vi "writePositionFirgelli.vi"(8 "error in (no error)":errorcluster, 9 "lengthMax":dbl=100.0, 10 "Position (mm)":dbl(slide)=1.0 min=0.0 max=100.0 step=0.1 scale=0.0..100.0 scale format="%.2f", 11 "handleIn":u32 format="%x") -> (0 "error out":errorcluster, 2 "regSetting":u16, 3 "handleOut":u32 format="%x")   [LabVIEW 2019]
doc: "0x20 SET_POSITION\nThis command allows USB control and disables RC, I, and V inputs until the system is rebooted. The data sent with this command determines what position the actuator moves too.\n\nFor example, to half way extend(25mm) a 50mm actuator, send 512. (The calculated value is rounded to a whole number).\n\nWritten by: Complete Automated Solutions\nwww.CompleteAutomatedSolutions.com"
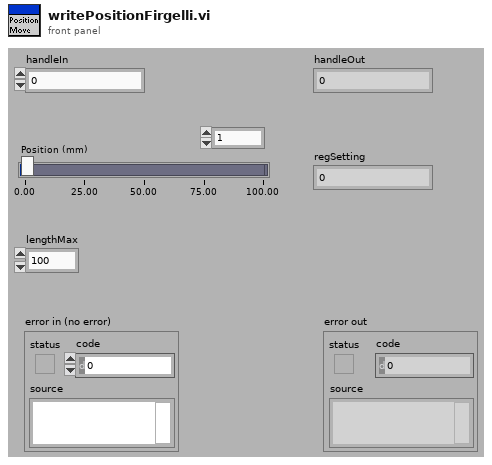
[diagram p1: front panel]
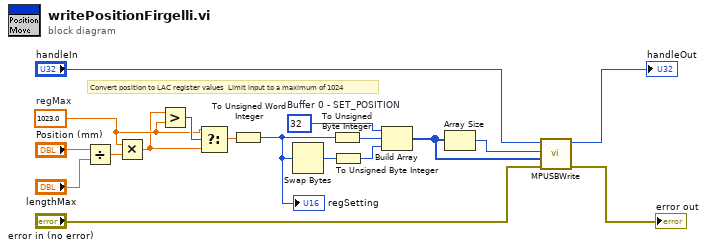
[diagram p0: block diagram]
diagram:
  w4 = 1023.0  # regMax
  w15 = u8 32  # Buffer 0 - SET_POSITION
  # "Convert position to LAC register values  Limit input to a maximum of 1024"
  n1 = Divide(x="Position (mm)", y="lengthMax") -> (x/y=w8:dbl)
  n2 = Multiply(x=w4, y=w8) -> (x*y=w3:dbl)
  n3 = Greater?(x=w3, y=w4) -> (0:w6:bool)
  n4 = Select(t=w4, s=w6, f=w3) -> (s? t:f=w2:dbl)
  n5 = To Unsigned Word Integer(number=w2) -> (unsigned 16bit integer=w1:u16)
  "regSetting" <- w1
  n6 = Swap Bytes(anything=w1) -> (byte swapped=w18:u16)
  n7 = To Unsigned Byte Integer(number=w1) -> (unsigned 8bit integer=w16:u8)
  n8 = To Unsigned Byte Integer(number=w18) -> (unsigned 8bit integer=w17:u8)
  n9 = Build Array(w15, w16, w17) -> (w13:u8[])
  n10 = Array Size(array=w13) -> (size(s)=w14:i32)
  n11 = call "MPUSBWrite.vi"("error in (no error)"="error in (no error)", "pDataIn"=w13, "dwLen"=w14, "handleIn"="handleIn") -> ("error out"=→"error out":errorcluster, "handleOut"=→"handleOut":u32)  [unwired: 2 in, 4 out]
